vi "ROI entry-check previous ROI Z plane range.vi"(7 "Z array size":i32, 8 "error in (no error)":errorcluster, 9 "Z value":dbl format="%#_13g", 10 "min Z":dbl, 11 "max Z":dbl) -> (0 "error out":errorcluster, 1 "Code":u8, 2 "Z plane Index":i32, 3 "Z value":dbl)   [LabVIEW 2020]
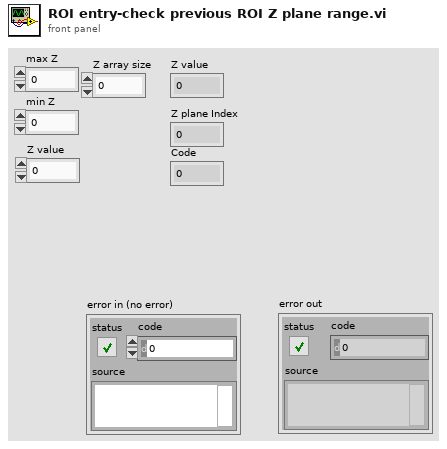
[diagram p1: front panel]
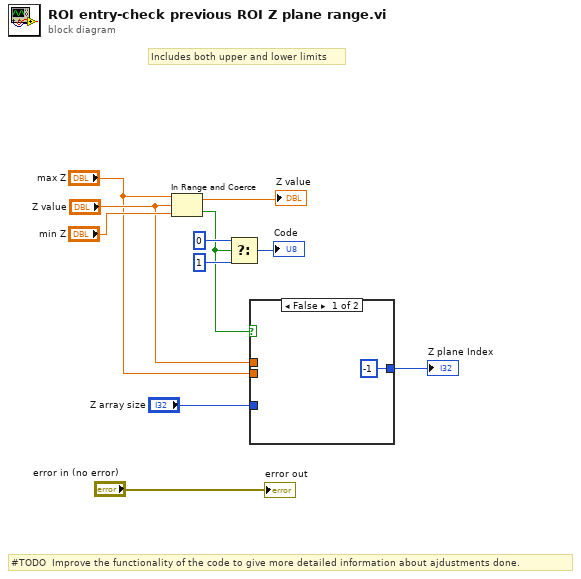
[diagram p0: block diagram]
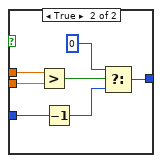
[diagram p2: hidden frame]
diagram:
  # "Includes both upper and lower limits"
  # "#TODO  Improve the functionality of the code to give more detailed information about ajdustments done."
  n1 = In Range and Coerce(upper limit="max Z", x="Z value", lower limit="min Z") -> (coerced(x)=→"Z value":dbl, In Range?=w5:bool)
  n2 = Select(t=u8 0, s=w5, f=u8 1 ("t")) -> (s? t:f=→"Code":u8)
  n3 = case shown="False" w5 {
    tunnel: "Z value" -> [_ w19]
    tunnel: "max Z" -> [_ w18]
    tunnel: "Z array size" -> [_ w15]
    tunnel: [-1 ("t") w13] -> w1
    frame False {
    }
    frame True {
      n4 = Greater?(x=w19, y=w18) -> (0:w17:bool)
      n5 = Decrement(x=w15) -> (x-1=w14:i32)
      n6 = Select(t=0, s=w17, f=w14) -> (s? t:f=w13:i32)
    }
  }
  "Z plane Index" <- w1
  "error out" <- "error in (no error)"
